vi "Get typeHistory.vi"(0 "Type":T1, 11 "error in (no error)":errorcluster) -> (8 "hsistory":string[][](array[string]), 14 "updated":bool, 15 "error out":errorcluster)   [LabVIEW 2011]
uses:
  emi Lib/System 01/0 - General/S&E reporting/Private/_emi_ S&E Message type.ctl
  E&S/Monitor/Actino S&E monitor.ctl
  E&S/String outpyt type.ctl
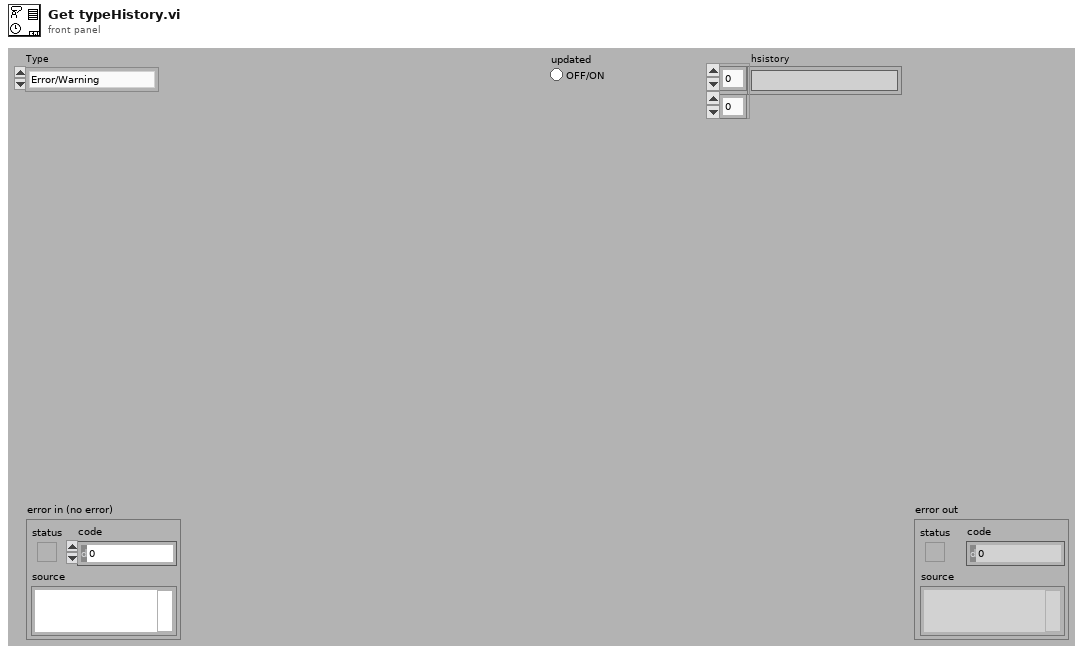
[diagram p1: front panel]
types:
  T1 = typedef "_emi_ S&E Message type.ctl" = enum16{"Error/Warning", "Note", "Debug", "Event", "Alarm Analog", "Alarm Digital", "Annotation"}
  T2 = typedef "Actino S&E monitor.ctl" = enum16{"GET(type history)", "SET S&E", "(Re)Init", "Get Error state", "Get  Alarm state", "Get All", "Get last  250", "Get Alarm History"}
  T3 = typedef "_emi_ S&E Message.ctl" = cluster{"Type":T1, "Originate time":dbl, "System":u8, "Loop":u16, "Sub ID":u16, "Elevated priority":bool, "E&S Message content":variant}
  T4 = typedef "String outpyt type.ctl" = enum16{"Full File hist", "Simple File hist", "Displ Hist one type", "Displ Hist mult types", "Displ Stat one type", "Displ Stat Mult type"}
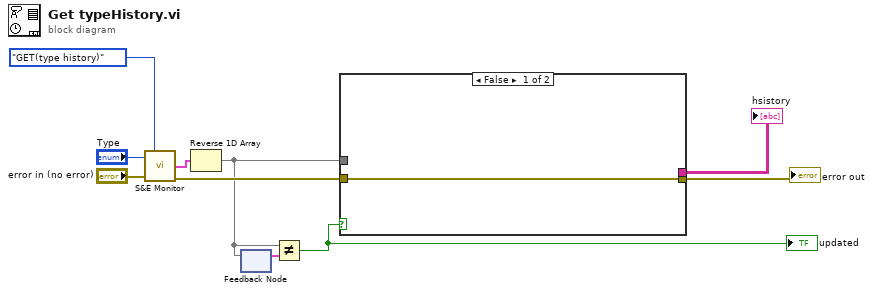
[diagram p0: block diagram]
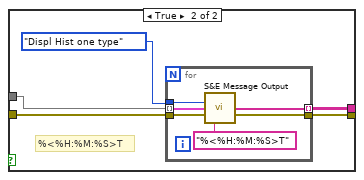
[diagram p2: hidden frame]
diagram:
  n1 = call "S&E Monitor.vi"("Action(GET 250)"=Actino_S&E_monitor."GET(type history)", "Type"="Type", "error in (no error)"="error in (no error)") -> ("S&E"=w8:T3[], "error out"=w5:errorcluster)  [unwired: 11 in]
  n2 = Reverse 1D Array(array=w8) -> (reversed array=w4:T3[])
  n3 = feedback-in #1(w4) -> ()
  n4 = feedback #1() -> (w7:T3[])  [unwired: 1 in]
  n5 = Not Equal?(x=w4, y=w7) -> (x != y?=w6:bool)
  "updated" <- w6
  n6 = case shown="False" w6 {
    tunnel: w5 -> [w11 w15]
    tunnel: w4 -> [_ w14]
    tunnel: [w11 w13] -> w2
    tunnel: [_ w12] -> w3
    frame False {
    }
    frame True {
      # "%<%H:%M:%S>T"
      n7 = for {
        tunnel: String_outpyt_type."Displ Hist one type" ("Type(File Hist)") -> [w22]
        tunnel: w15 -> [w21]
        tunnel: w14 -> [w20] mode=indexing
        tunnel: [w19] -> w13
        tunnel: [w17] -> w12 mode=indexing
        n8 = call "S&E Message Output.vi"("Type(File Hist)"=w22, "E&S Message"=w20, "error in (no error)"=w21, "Time format(%T)"="%<%H:%M:%S>T") -> ("Array of strings"=w17:string[], "error out"=w19:errorcluster)  [unwired: 9 in, 1 out]
      }
    }
  }
  "error out" <- w2
  "hsistory" <- w3
